vi "Teardown.vi"(7 "Sender":refnum<class "Sender.lvclass">, 11 "Teardown in":refnum<class "Teardown.lvclass">) -> (3 "Teardown out":refnum<class "Teardown.lvclass">)   [LabVIEW 2020, in "jettl.lvlib" / "Teardown Msg.lvlib" / "Teardown.lvclass"]
uses:
  Teardown.lvclass
  Sender/Sender/Sender.lvclass
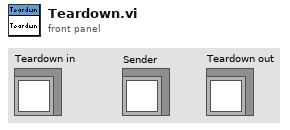
[diagram p1: front panel]
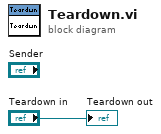
[diagram p0: block diagram]
diagram:
  "Teardown out" <- "Teardown in"
